vi "TOOLweb CAPABILITIES.vi"(4 "error in (no error)":errorcluster caption="Fehler (Eingang, kein Fehler)", 5 "IP-Adresse (localhost)":string="127.0.0.1") -> (0 "error out":errorcluster caption="Fehler (Ausgang)", 3 "Capabilities":string)   [LabVIEW 2020, in "FT-IR.lvlib" / "TOOLweb Interface.lvlib"]
doc: "Holt Informationen über verfügbare Befehle, EVID-Nummern, Formate und Datentypen vom Messgerät ( Discovery Handshake).\n\nFalls der TOOLWeb-Server nicht auf demselben Rechner arbeitet, kann mit \"IP-Adresse\" eine beliebiger Host adressiert werden. Ein unverbundener Eingang spricht den lokalen Host an."
uses:
  TOOLweb Interface.lvlib
  TOOLweb Interface Hilfs-VIs.lvlib
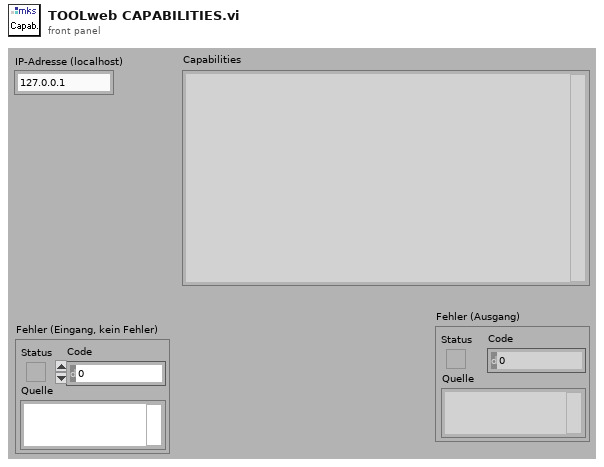
[diagram p1: front panel]
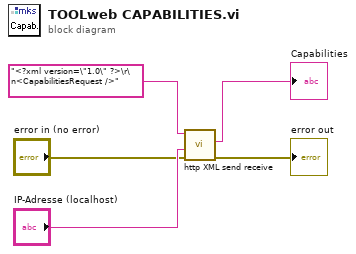
[diagram p0: block diagram]
diagram:
  n1 = call "http XML send receive.vi"("error in (no error)"="error in (no error)", "IP-Adresse (localhost)"="IP-Adresse (localhost)", "XML Request"="<?xml version=\"1.0\" ?>\r\n<CapabilitiesRequest />" ("Daten (Eingang)")) -> ("error out"=→"error out":errorcluster, "Response Body (XML)"=→"Capabilities":string)  [unwired: 3 out]
